vi "Conveyer Belt Move Control.vi"(1 "Conveyer Belt Information In":T1) -> (0 "Conveyer Belt Information Out":T1)   [LabVIEW 2012]
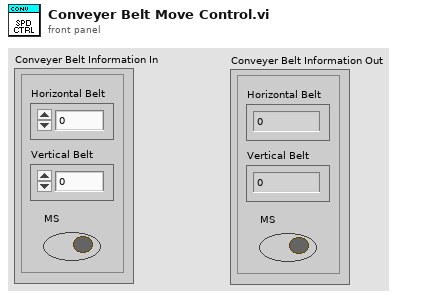
[diagram p1: front panel]
types:
  T1 = cluster{"Horizontal Belt":dbl, "Vertical Belt":dbl, "MS":bool}
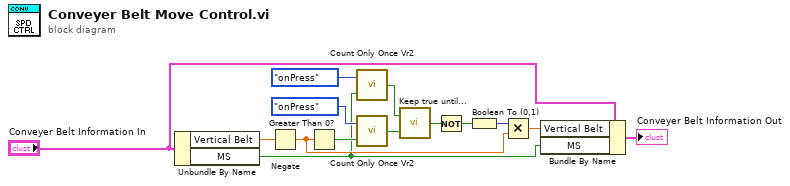
[diagram p0: block diagram]
diagram:
  n1 = Unbundle By Name("Conveyer Belt Information In") -> ("Vertical Belt"=w12:dbl, "MS"=w1:bool)
  n2 = Negate(x=w12) -> (-x=w3:dbl)
  n3 = Greater Than 0?(x=w3) -> (x > 0?=w9:bool)
  n4 = call "Count Only Once Vr2.vi"("InValue"=w1, "Action"=enum16{"onPress", "onRelease", "Both"}."onPress") -> ("Result"=w8:bool)
  n5 = call "Count Only Once Vr2.vi"("InValue"=w9, "Action"=enum16{"onPress", "onRelease", "Both"}."onPress") -> ("Result"=w7:bool)
  n6 = call "Keep true until....vi"("Changer"=w7, "Keep"=w8) -> ("Value"=w6:bool)
  n7 = Not(x=w6) -> (.not. x?=w5:bool)
  n8 = Boolean To (0,1)(Boolean=w5) -> (0, 1=w4:i16)
  n9 = Multiply(x=w4, y=w3) -> (x*y=w2:dbl)
  n10 = Bundle By Name(cluster="Conveyer Belt Information In", "Vertical Belt"=w2, "MS"=w1) -> (→"Conveyer Belt Information Out":T1)
